vi "Initial Systems.vi"() -> (0 "Magnet 2":T1=enum."Cell8", 1 "Data Acq 2":T2=enum."NML Data Acquisition-New.vi")   [LabVIEW 2019]
uses:
  Ctl/Data Acquisition System.ctl
  Ctl/magnet.ctl
panel:
  in  "enter":bool
  in  "Magnet":T1=enum."SCM2"
  in  "Data Acq":T2=enum."NML Data Acquisition-New.vi"
  # "Select your Data Acquisition System"
  # "Select your Magnet System"
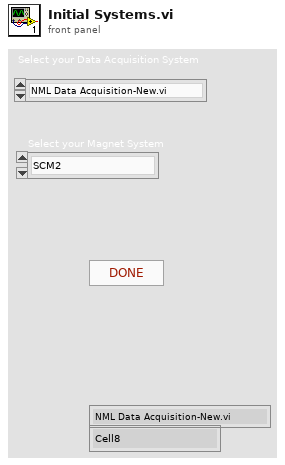
[diagram p1: front panel]
types:
  T1 = typedef "magnet.ctl" = enum16{"SCM1", "SCM2", "SCM3", "SCMX", "Cell8", "Cell9", "Cell12", "Hybrid", "Great Magnet"}
  T2 = typedef "Data Acquisition System.ctl" = enum16{"NML Data Acquisition-old.vi", "NML Data Acquisition-New.vi"}
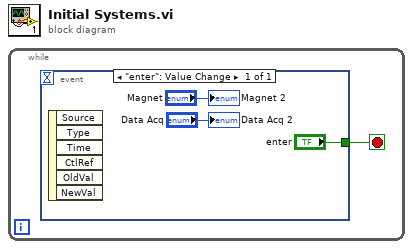
[diagram p0: block diagram]
diagram:
  n1 = while {
    stop <- w1 stop-if-true
    n2 = event shown="[0] \"enter\": Value Change" {
      selector: _ -> [_]
      dyn-events: _ -> [_]
      timeout: _ -> [_]
      tunnel: ["enter"] -> w1
      event "enter": Value Change {
        n3 = event-data() -> ()  [unwired: 1 in, 6 out]
        "Data Acq 2" <- "Data Acq"
        "Magnet 2" <- "Magnet"
      }
    }
  }
